vi "predictTrajectory.vi"() -> ()   [LabVIEW 2014]
panel:
  in  "percentage threshold of energy remained for the cannonball not bouncing again":dbl=30.0 format="%#_g%"
  in  "percentage of energy loss":dbl=30.0 format="%#_g%"
  in  "initial angle":dbl=60.0 format="%#_g°"
  in  "initial velocity":dbl=10.0 format="%#_gm/s"
  out "percentage threshold":dbl
  out "initial v":dbl
  out "?":bool
  # "from here"
  # "程式第一次跑好像會錯誤@@"
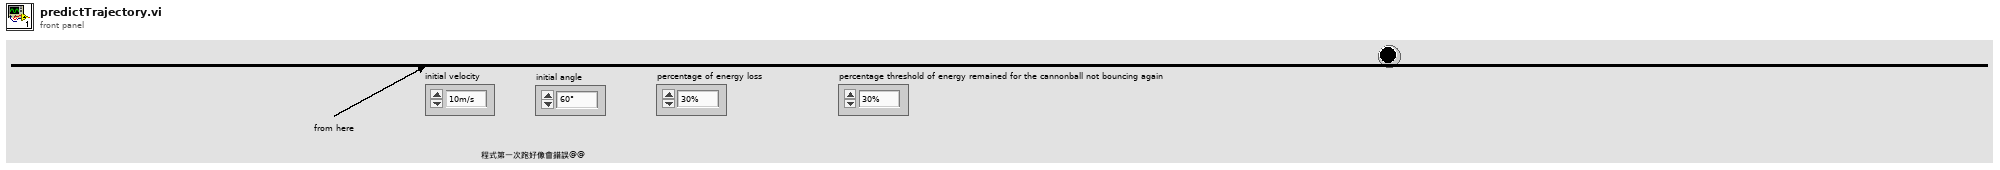
[diagram p1: front panel]
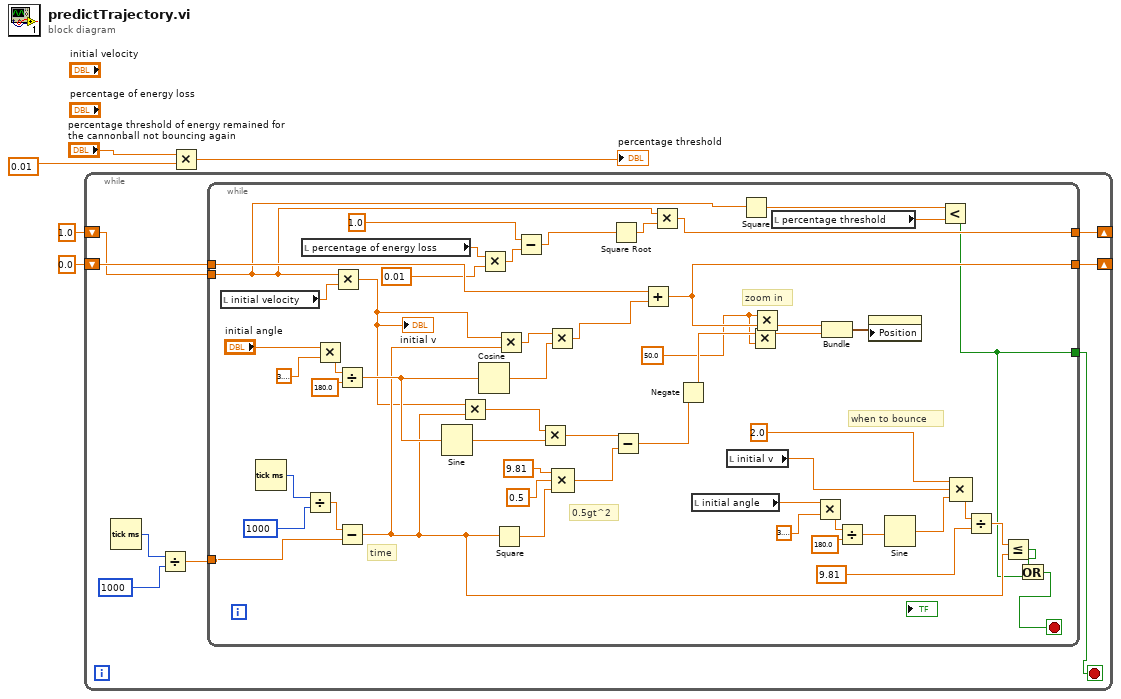
[diagram p0: block diagram]
diagram:
  n1 = while {
    shift-right: [w9] -> _
    shift-left: 0.0 -> [w10]
    shift-right: [w8] -> _
    shift-left: 1.0 -> [w7]
    stop <- w6 stop-if-true
    n2 = Tick Count (ms)() -> (millisecond timer value=w13:u32)
    n3 = Divide(x=w13, y=1000) -> (x/y=w11:dbl)
    n4 = while {
      tunnel: w11 -> [w64]
      tunnel: w10 -> [w38]
      tunnel: [w36] -> w9
      tunnel: [w30] -> w8
      tunnel: w7 -> [w25]
      tunnel: [w21] -> w6
      stop <- w20 stop-if-true
      w26 = 50.0
      # "0.5gt^2"
      # "time"
      # "when to bounce"
      # "zoom in"
      n5 = local read "initial velocity"() -> (w14:dbl)
      n6 = Tick Count (ms)() -> (millisecond timer value=w67:u32)
      n7 = local read "percentage of energy loss"() -> (w15:dbl)
      n8 = Divide(x=w67, y=1000) -> (x/y=w65:dbl)
      n9 = Multiply(x="initial angle", y=3.141592653589793) -> (x*y=w60:dbl)
      n10 = Multiply(x=w25, y=w14) -> (x*y=w16:dbl)
      "initial v" <- w16
      n11 = Divide(x=w60, y=180.0) -> (x/y=w57:dbl)
      n12 = Subtract(x=w65, y=w64) -> (x-y=w42:dbl)
      n13 = Sine(x=w57) -> (sin(x)=w54:dbl)
      n14 = Multiply(x=w16, y=w42) -> (x*y=w50:dbl)
      n15 = Cosine(x=w57) -> (cos(x)=w63:dbl)
      n16 = Multiply(x=w15, y=0.01) -> (x*y=w33:dbl)
      n17 = Square(x=w42) -> (x^2=w52:dbl)
      n18 = Multiply(x=w16, y=w42) -> (x*y=w49:dbl)
      n19 = Subtract(x=1.0, y=w33) -> (x-y=w32:dbl)
      n20 = Multiply(x=w50, y=w54) -> (x*y=w62:dbl)
      n21 = Multiply(x=w49, y=w63) -> (x*y=w37:dbl)
      n22 = Compound Arithmetic op=MULTIPLY(9.81, 0.5, w52) -> (w55:dbl)
      n23 = Square Root(x=w32) -> (sqrt(x)=w31:dbl)
      n24 = Subtract(x=w62, y=w55) -> (x-y=w48:dbl)
      n25 = Add(x=w38, y=w37) -> (x+y=w36:dbl)
      n26 = Multiply(x=w25, y=w31) -> (x*y=w30:dbl)
      n27 = Negate(x=w48) -> (-x=w53:dbl)
      n28 = local read "initial angle"() -> (w17:dbl)
      n29 = local read "initial v"() -> (w29:dbl)
      n30 = Square(x=w25) -> (x^2=w24:dbl)
      n31 = Multiply(x=w53, y=w26) -> (x*y=w27:dbl)
      n32 = Multiply(x=w26, y=w36) -> (x*y=w28:dbl)
      n33 = local read "percentage threshold"() -> (w23:dbl)
      n34 = Multiply(x=w17, y=3.141592653589793) -> (x*y=w47:dbl)
      n35 = Bundle(w28, w27) -> (w51:cluster{dbl, dbl})  [unwired: 1 in]
      n36 = Divide(x=w47, y=180.0) -> (x/y=w41:dbl)
      n37 = property class="Bool (strict)"("Position"=w51) -> ()  [unwired: 2 in, 2 out]
      n38 = Sine(x=w41) -> (sin(x)=w40:dbl)
      n39 = Less?(x=w24, y=w23) -> (x < y?=w21:bool)
      n40 = Compound Arithmetic op=MULTIPLY(2.0, w29, w40) -> (w44:dbl)
      n41 = Divide(x=w44, y=9.81) -> (x/y=w39:dbl)
      n42 = Less Or Equal?(x=w39, y=w42) -> (x <= y?=w22:bool)
      n43 = Or(x=w22, y=w21) -> (x .or. y?=w20:bool)
    }
  }
  n44 = Multiply(x="percentage threshold of energy remained for the cannonball not bouncing again", y=0.01) -> (x*y=→"percentage threshold":dbl)
